vi "table2bd.vi"(3 "error in (no error)":errorcluster, 4 "eeert":string[][](table)=[["", "Фаза", "Ch0", "6", "Градусы"], ["", "Фаза", "Ch1", "7", "Градусы"], ["", "Фаза", "Ch2", "1", "Градусы"], ["", "Фаза", "Ch3", "2", "Градусы"], ["", "Фаза", "Ch4", "3", "Градусы"], ["", "Напряжение/Ток", "Ch0", "0,00", "В"], ["", "Напряжение/Ток", "Ch1", "0,00", "В"], ["", "Напряжение/Ток", "Ch2", "0,00", "В"], ["", "Напряжение/Ток", "Ch3", "0,00", "В"], ["", "Напряжение/Ток", "Ch4", "0,00", "В"], ["", "Частота", "Ch0", "300,00", "Гц"]], 5 "time stamp":timestamp) -> (0 "error out":errorcluster)   [LabVIEW 2010]
uses:
  <vilib>/addons/database/Auxilliary.llb/DB Tools Column Info.ctl
  <vilib>/addons/database/Auxilliary.llb/DB Tools DataTypes.ctl
  70user.lib/TheSigTab.vi
  <vilib>/addons/database/NI_Database_API.lvlib
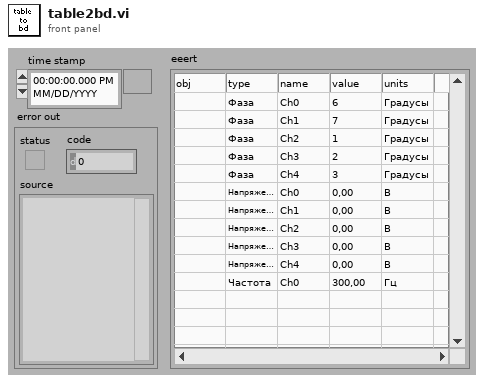
[diagram p1: front panel]
types:
  T1 = cluster{"type":string, "name":string, "val":dbl, "units":string, "sig_id":i32, "date_time":string, "Obj_Id":i32}
  T2 = typedef "NI_Database_API.lvlib/DB Tools Column Info.ctl" = cluster{"column name":string, "data type":T3, "size":i32, "allow null?":bool}
  T3 = typedef "NI_Database_API.lvlib/DB Tools DataTypes.ctl" = enum16{"String", "Long (I32)", "Single (SGL)", "Double (DBL)", "Date/Time", "Binary"}
  T4 = typedef "NI_Database_API.lvlib/Conn ObjectReference.ctl" = refnum<k1>
  T5 = cluster{"eeert[0]":string, "eeert[1]":string, "eeert[2]":string, "eeert[3]":string, "eeert[4]":string}
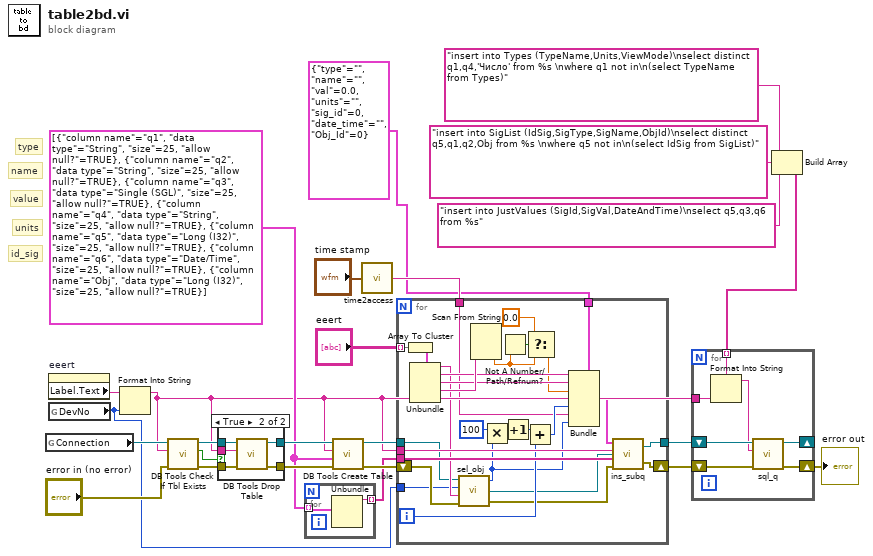
[diagram p0: block diagram]
diagram:
  w19 = T2[] [{"column name"="q1", "data type"=enum."String", "size"=25, "allow null?"=TRUE}, {"column name"="q2", "data type"=enum."String", "size"=25, "allow null?"=TRUE}, {"column name"="q3", "data type"=enum."Single (SGL)", "size"=25, "allow null?"=TRUE}, {"column name"="q4", "data type"=enum."String", "size"=25, "allow null?"=TRUE}, {"column name"="q5", "data type"=enum."Long (I32)", "size"=25, "allow null?"=TRUE}, {"column name"="q6", "data type"=enum."Date/Time", "size"=25, "allow null?"=TRUE}, {"column name"="Obj", "data type"=enum."Long (I32)", "size"=25, "allow null?"=TRUE}]
  # "value"
  # "name"
  # "id_sig"
  # "units"
  # "type"
  n1 = global read "TheSigTab.vi" "Connection"() -> (w13:T4)
  n2 = property on="eeert" class="Tbl (strict)"() -> ("Label.Text"=w18:string)  [unwired: 2 in, 2 out]
  n3 = global read "TheSigTab.vi" "DevNo"() -> (w2:u32)
  n4 = Format Into String(initial string=w18, w2) -> (resulting string=w12:string)  [unwired: 2 in, 1 out]
  n5 = call <vilib>:"DB Tools Check If Tbl Exists.vi"("error in (no error)"="error in (no error)", "table name"=w12, "connection reference"=w13) -> ("error out"=w14:errorcluster, "exists?"=w16:bool, "connection reference out"=w15:T4)  [unwired: 2 in]
  n6 = case shown="True" w16 {
    tunnel: [w27 w32] -> w25
    tunnel: w12 -> [_ w31]
    tunnel: [w26 w30] -> w22
    tunnel: w15 -> [w27 w29]
    tunnel: w14 -> [w26 w28]
    frame False {
    }
    frame True {
      n7 = call <vilib>:"DB Tools Drop Table.vi"("error in (no error)"=w28, "table"=w31, "connection reference"=w29) -> ("error out"=w30:errorcluster, "connection reference out"=w32:T4)  [unwired: 5 in]
    }
  }
  n8 = for {
    tunnel: w19 -> [w34] mode=indexing
    tunnel: [w33] -> w17 mode=indexing
    n9 = Unbundle(w34) -> ("column name"=w33:string)  [unwired: 3 out]
  }
  n10 = call <vilib>:"DB Tools Create Table.vi"("error in (no error)"=w22, "column information"=w19, "table"=w12, "connection reference"=w25) -> ("error out"=w23:errorcluster, "connection reference out"=w24:T4)  [unwired: 4 in]
  n11 = call "time2access.vi"("time stamp"="time stamp") -> ("date/time string"=w21:string)
  n12 = for {
    tunnel: [w62] -> w8
    tunnel: w12 -> [w61]
    tunnel: w24 -> [w49]
    tunnel: w17 -> [w60]
    tunnel: "eeert" -> [w59] mode=indexing
    shift-right: [w63] -> w9
    shift-left: w23 -> [w47]
    tunnel: w21 -> [w42]
    tunnel: w2 -> [w36]
    tunnel: T1 {"type"="", "name"="", "val"=0.0, "units"="", "sig_id"=0, "date_time"="", "Obj_Id"=0} ("anything") -> [w35]
    i -> [w57]
    n13 = Array To Cluster(array=w59) -> (cluster=w56:T5)
    n14 = Unbundle(w56) -> ("eeert[0]"=w50:string, "eeert[1]"=w51:string, "eeert[2]"=w52:string, "eeert[3]"=w53:string, "eeert[4]"=w54:string)
    n15 = call "sel_obj.vi"("error in"=w47, "Object"=w50, "DevNo"=w36, "conn ref in"=w49) -> ("error out"=w46:errorcluster, "conn ref out"=w48:T4, "Obj Id"=w37:i32)
    n16 = Scan From String(input string=w53) -> (output 1=w40:dbl)  [unwired: 4 in, 3 out]
    n17 = Multiply(x=100, y=w37) -> (x*y=w45:i32)
    n18 = Not A Number/Path/Refnum?(number/path/refnum=w40) -> (NaN/Path/Refnum?=w41:bool)
    n19 = Increment(x=w45) -> (x+1=w43:i32)
    n20 = Add(x=w43, y=w57) -> (x+y=w55:i32)
    n21 = Select(t=0.0, s=w41, f=w40) -> (s? t:f=w38:dbl)
    n22 = Bundle(cluster=w35, "type"=w51, "name"=w52, "val"=w38, "units"=w54, "sig_id"=w55, "date_time"=w42, "Obj_Id"=w37) -> (w58:T1)
    n23 = call "ins_subq.vi"("data"=w58, "table_name"=w61, "columns"=w60, "error out"=w46, "conn ref out"=w48) -> ("connection reference out"=w62:T4, "error out 2"=w63:errorcluster)
  }
  n24 = Build Array("insert into Types (TypeName,Units,ViewMode)\nselect distinct q1,q4,'Число' from %s \nwhere q1 not in\n(select TypeName from Types)" ("optional clause"), "insert into SigList (IdSig,SigType,SigName,ObjId)\nselect distinct q5,q1,q2,Obj from %s \nwhere q5 not in\n(select IdSig from SigList)", "insert into JustValues (SigId,SigVal,DateAndTime)\nselect q5,q3,q6 from %s") -> (w3:string[])
  n25 = for {
    tunnel: w12 -> [w70]
    shift-right: [w65] -> _
    shift-left: w8 -> [w68]
    shift-right: [w66] -> w4
    shift-left: w9 -> [w69]
    tunnel: w3 -> [w64] mode=indexing
    n26 = Format Into String(format string=w64, w70) -> (resulting string=w67:string)  [unwired: 2 in, 1 out]
    n27 = call "sql_q.vi"("error in"=w69, "SQL query"=w67, "connect ref"=w68) -> ("error out"=w66:errorcluster, "conn ref out"=w65:T4)  [unwired: 1 in, 2 out]
  }
  "error out" <- w4
